vi "Test_ExecuteCalibration.vi"() -> ()   [LabVIEW 2019]
uses:
  ByteGSAPIBase/CalibrationMeasurements/BodyCalibrazioneMisure.ctl
  ByteGSAPIBase/FetchCalibration/Converted_Slug_Cluster.ctl
  ByteGSAPIBase/ByteGSAPIBase.lvclass
  <vilib>/DAQmx/write.llb/DAQmx Write (Analog DBL 1Chan 1Samp).vi
  <vilib>/DAQmx/read.llb/DAQmx Read (Analog DBL 1Chan 1Samp).vi
  2f0a0fb9-248b-477a-8bd2-6224b53458e2.vi
  <vilib>/DAQmx/create/channels.llb/DAQmx Create Channel (AI-Voltage-Basic).vi
  <vilib>/DAQmx/create/channels.llb/DAQmx Create Channel (AO-Voltage-Basic).vi
  <vilib>/DAQmx/miscellaneous.llb/DAQmx Fill In Error Info.vi
  <vilib>/Bytelabs/ByteSimpleQ/ByteSimpleQ/ByteSimpleQ.lvlib
panel:
  in  "Exit":bool
  in  "Calibrate":bool
  in  "Btn-Start-Oriz":bool
  in  "DueDateInstruments":i32(listbox)
  out "Waveform Chart":dbl(graph)
  out "logical AND":bool
  out "Mpe_min":dbl format="%.3f"
  out "Mpe_Max":dbl format="%.3f"
  out "Temp":sgl format="%.1f °C"
  out "Hr%":sgl format="%.1f Hr%"
  out "nmisure":u32 format="# %d"
  out "UoM":string
  out "Measure":dbl format="%0.2f"
  out "measurement_group_passed":u32(colorbox)
  in  "SetPoint":dbl format="%0.2f"
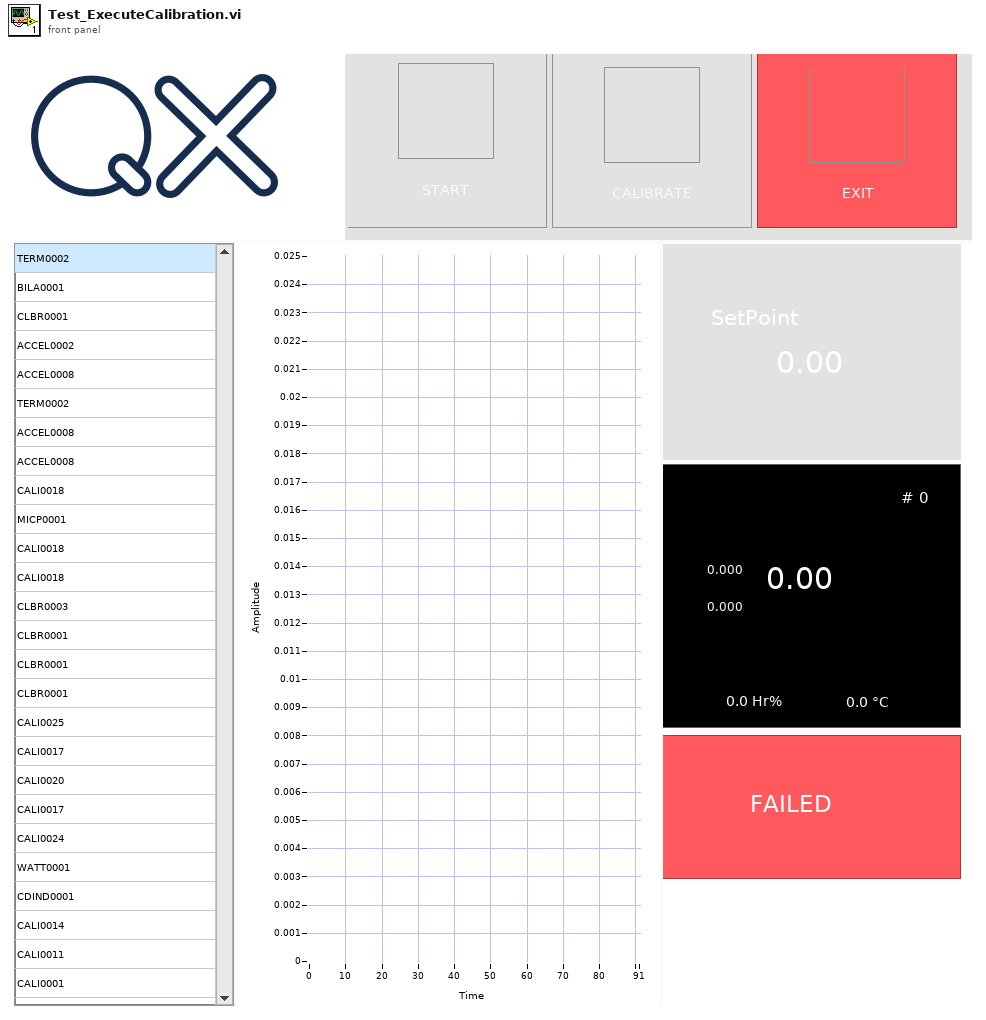
[diagram p1: front panel]
types:
  T1 = typedef "ByteGSWebAPI.lvlib/ByteGSAPIBase.lvclass/BodyCalibrazioneMisure.ctl" = cluster{"controls":cluster{"id":u16, "descrizione":string, "numero_misure_necessarie":u16, "riferimento_obiettivo":dbl, "mpe_max":dbl, "mpe_min":dbl, "deviazione_standard":dbl, "incertezza":dbl, "numero_misure_effettuate":u32, "temperatura_c":dbl, "umidita":dbl, "strumento_riferimento":cluster{"id":u16, "nome":string}[]}[]}
  T2 = typedef "ByteGSWebAPI.lvlib/ByteGSAPIBase.lvclass/Converted_Slug_Cluster.ctl" = cluster{"id":u32, "instrument":string, "name":string, "date":timestamp}
  T3 = cluster{"AI":refnum<k21>, "AO":refnum<k21>, "IdInstrument":i32[], "Calibration data":T1, "Measure":dbl, "idFailed":u32, "passed":bool, "Read?":bool, "CalibIndex":i32, "TotMeasure":i32, "riferimento_obiettivo":dbl, "ExpiredInstruments":T2[]}
  T4 = enum8{"Enabled", "Disabled", "Disabled and Grayed Out"}
  T5 = typedef "Instruments.ctl" = cluster{"id":i32, "slug":string, "stabilimento":cluster{"id":dbl}, "categoria":cluster{"id":dbl}, "tipologia_di_visualizzazione":cluster{"id":dbl}, "stato":cluster{"id":dbl}, "descrizione":string, "costruttore":string, "matricola":string, "data_registrazione":string, "intervallo_di_taratura_mesi":dbl, "reparto":string, "campo_misura":string, "risoluzione":dbl, "responsabile_strumento":string, "classe_di_precisione":string, "classificazione":string, "appunti":string, "manuale":string, "foto":string, "riferimento":bool, "qr_hashcode":string, "costo_euro":dbl}
  T6 = cluster{"id":u16, "descrizione":string, "numero_misure_necessarie":u16, "riferimento_obiettivo":dbl, "mpe_max":dbl, "mpe_min":dbl, "deviazione_standard":dbl, "incertezza":dbl, "numero_misure_effettuate":u32, "temperatura_c":dbl, "umidita":dbl, "strumento_riferimento":cluster{"id":u16, "nome":string}[]}[]
  T7 = cluster{"id":u16, "descrizione":string, "numero_misure_necessarie":u16, "riferimento_obiettivo":dbl, "mpe_max":dbl, "mpe_min":dbl, "deviazione_standard":dbl, "incertezza":dbl, "numero_misure_effettuate":u32, "temperatura_c":dbl, "umidita":dbl, "strumento_riferimento":cluster{"id":u16, "nome":string}[]}
  T8 = cluster{"id":u32, "control_id":u32, "passed":bool}[]
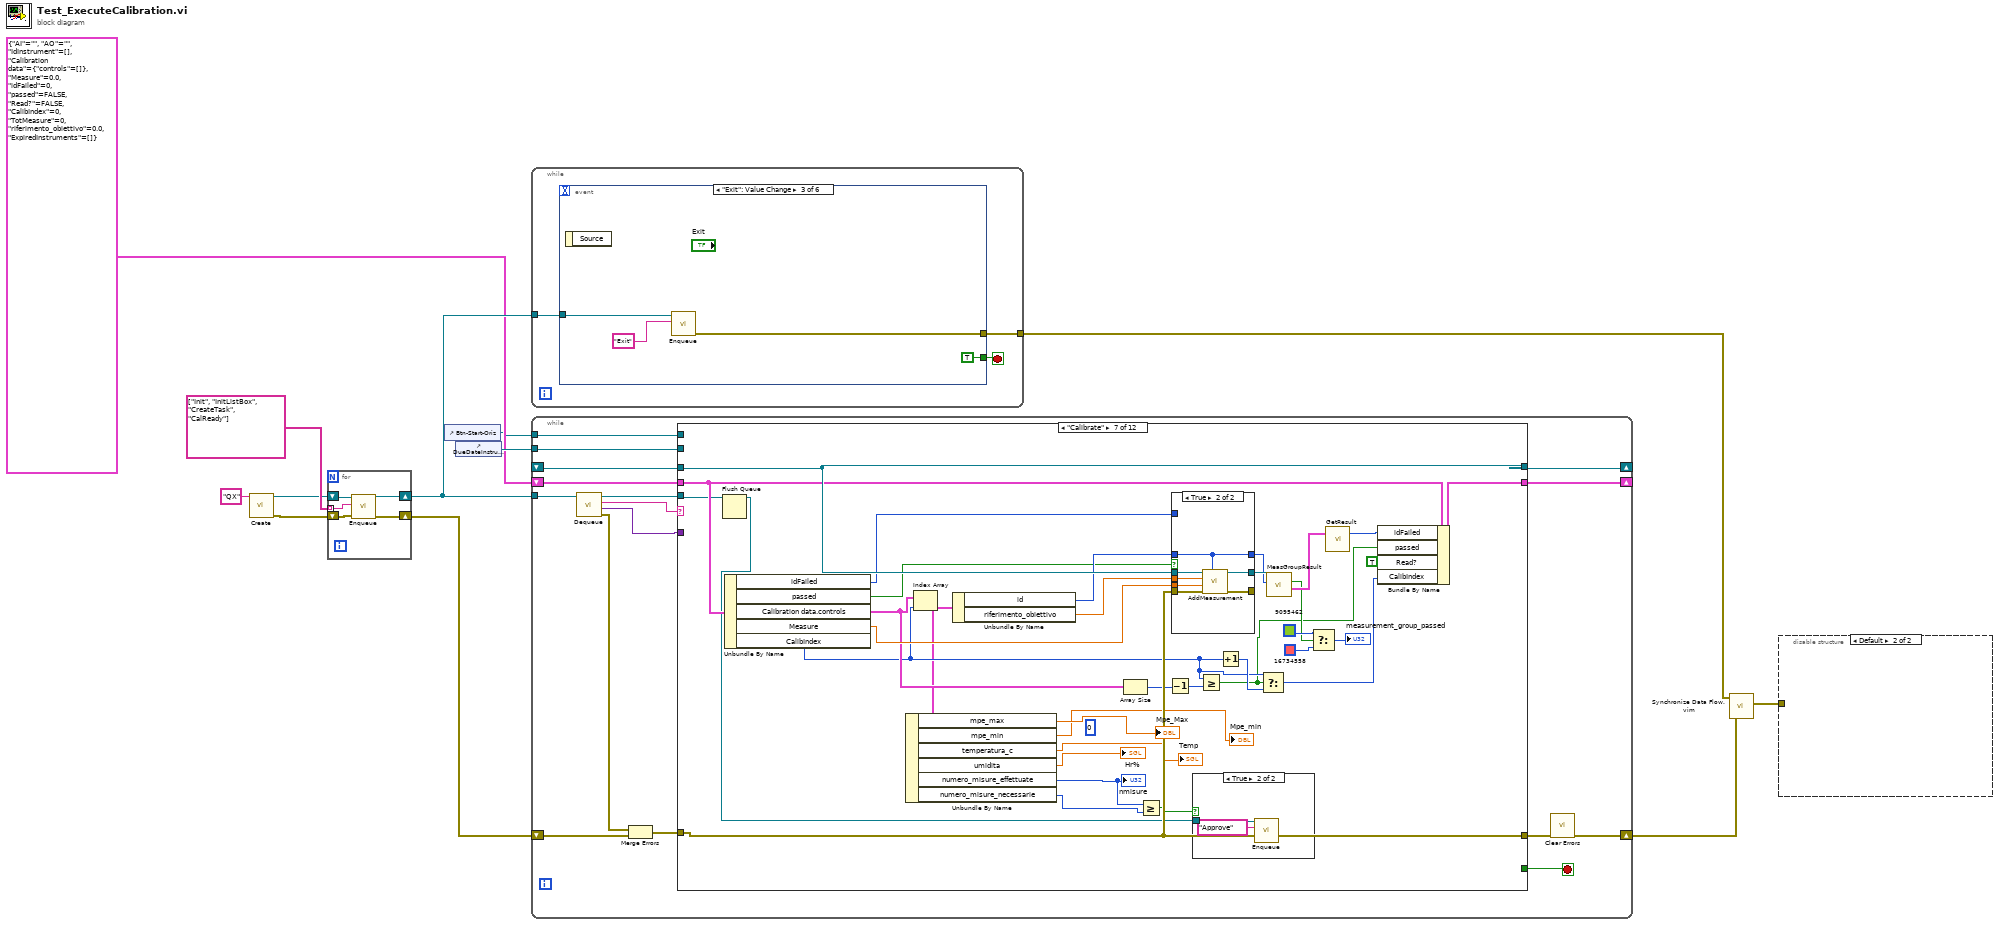
[diagram p0: block diagram]
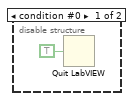
[diagram p2: hidden frame]
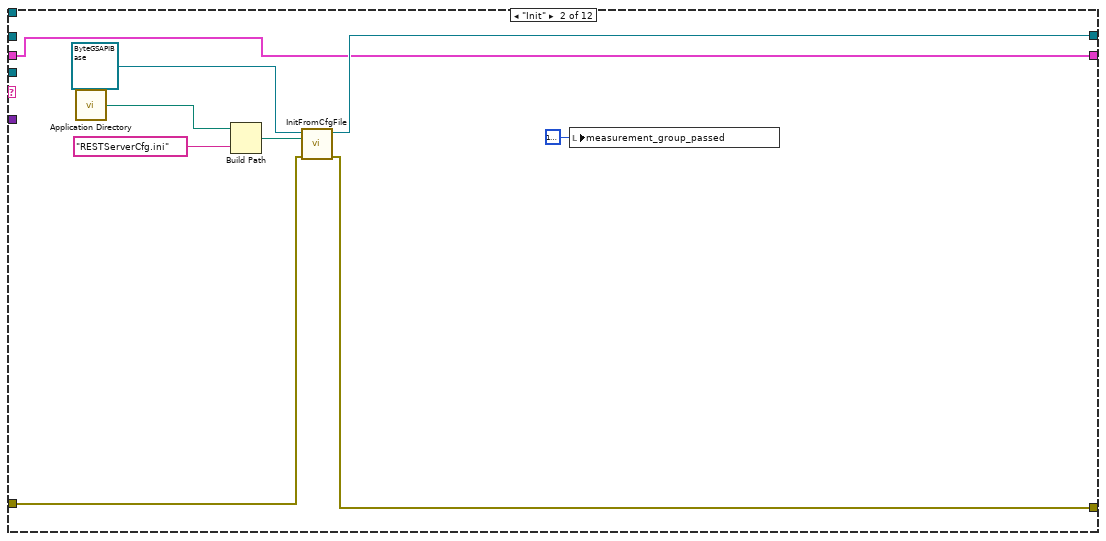
[diagram p4: hidden frame]
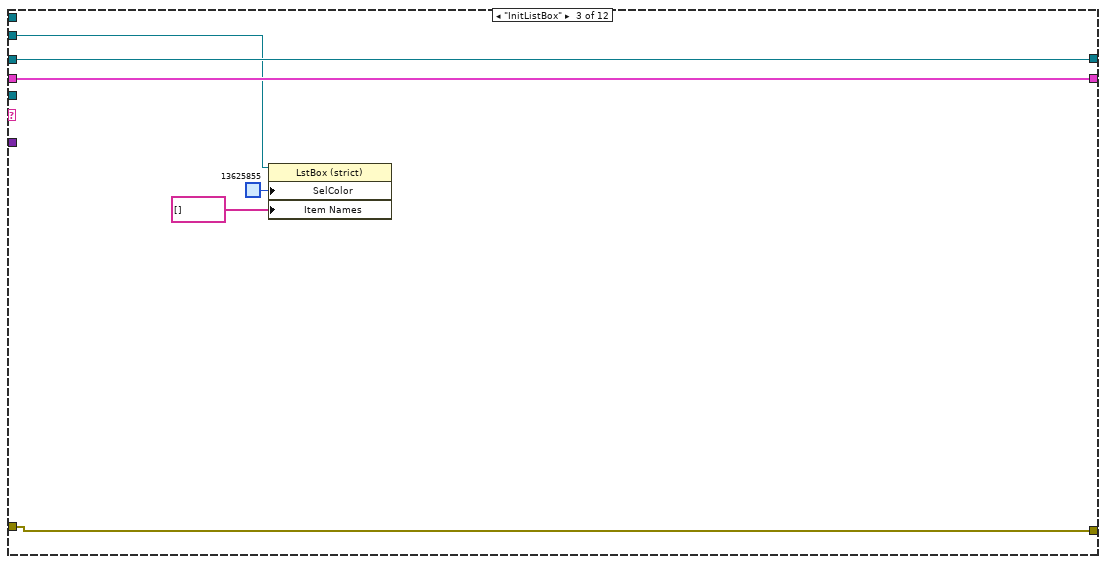
[diagram p5: hidden frame]
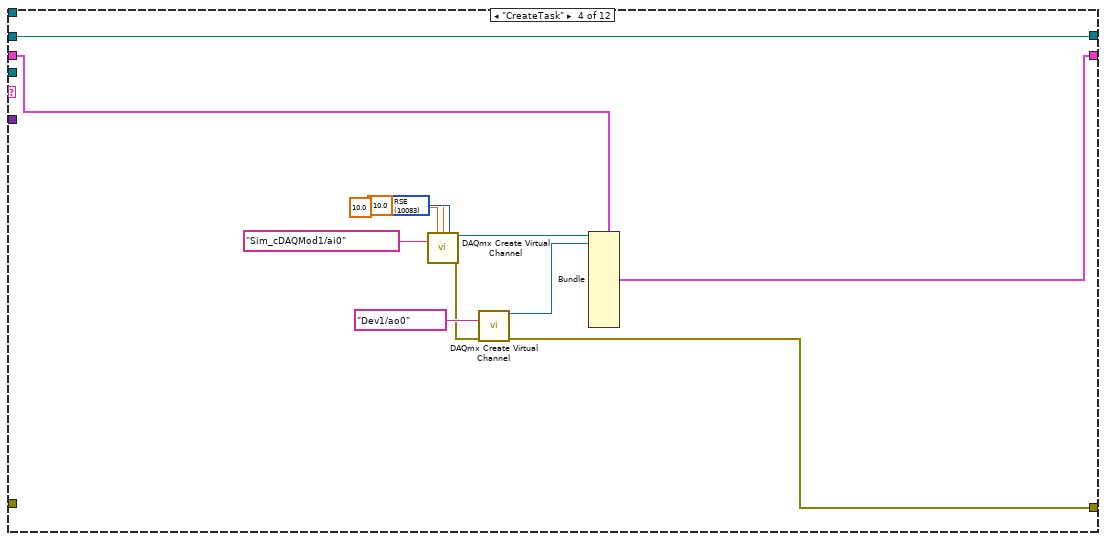
[diagram p6: hidden frame]
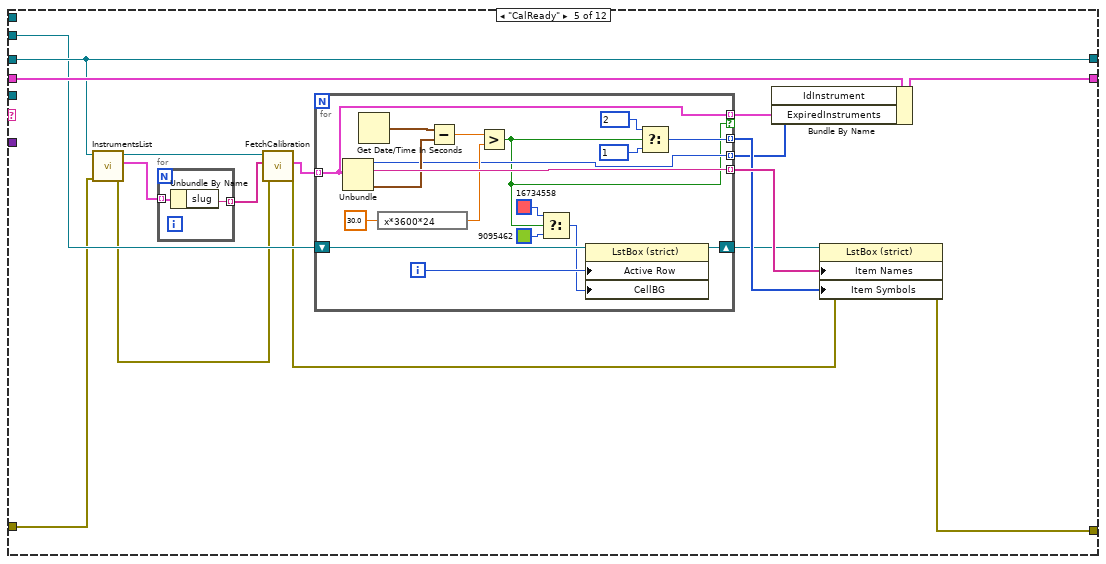
[diagram p7: hidden frame]
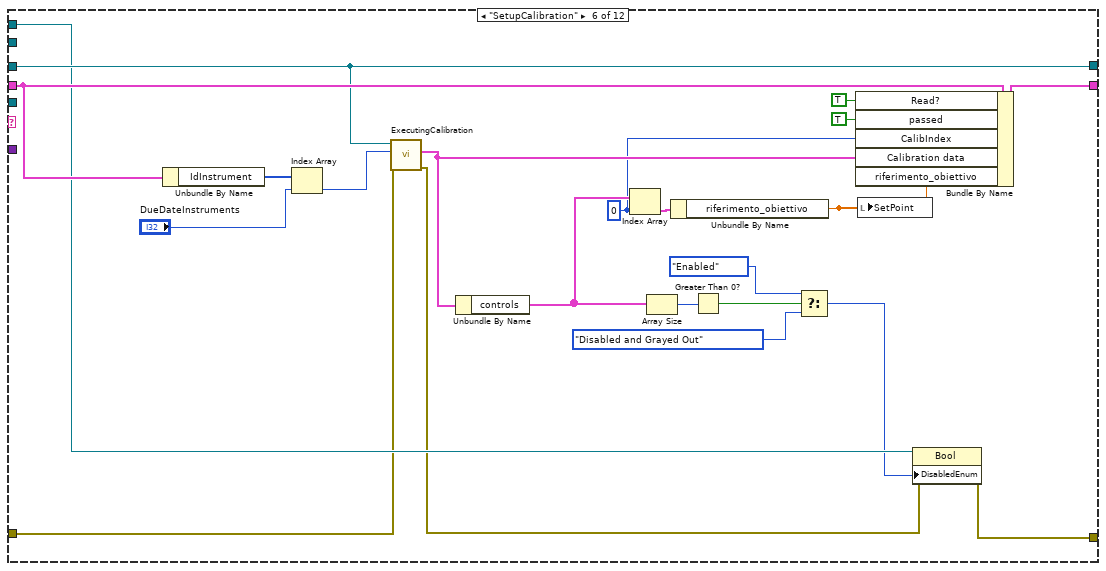
[diagram p8: hidden frame]
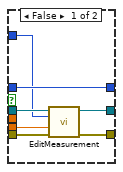
[diagram p10: hidden frame]
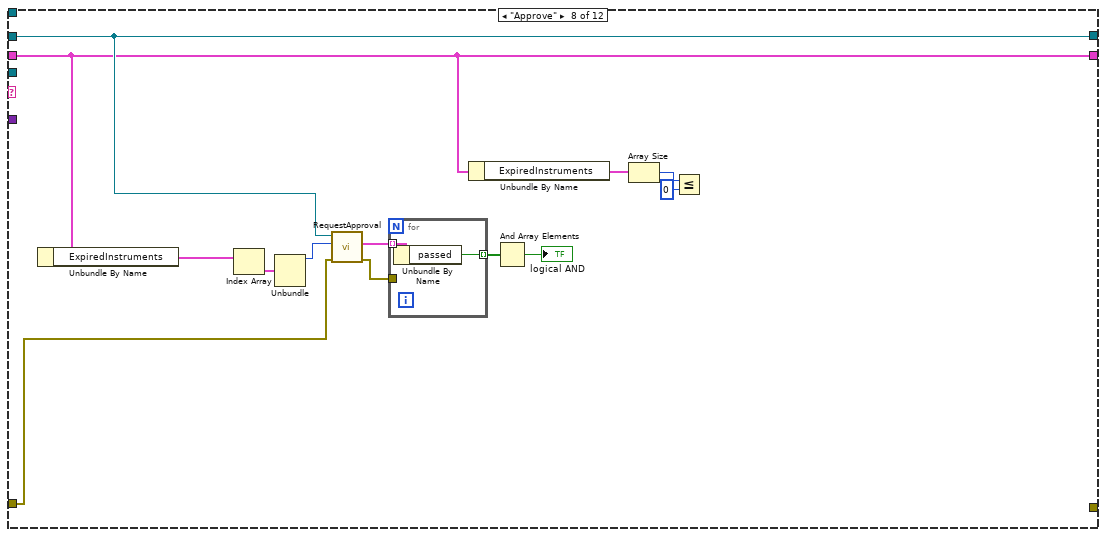
[diagram p11: hidden frame]
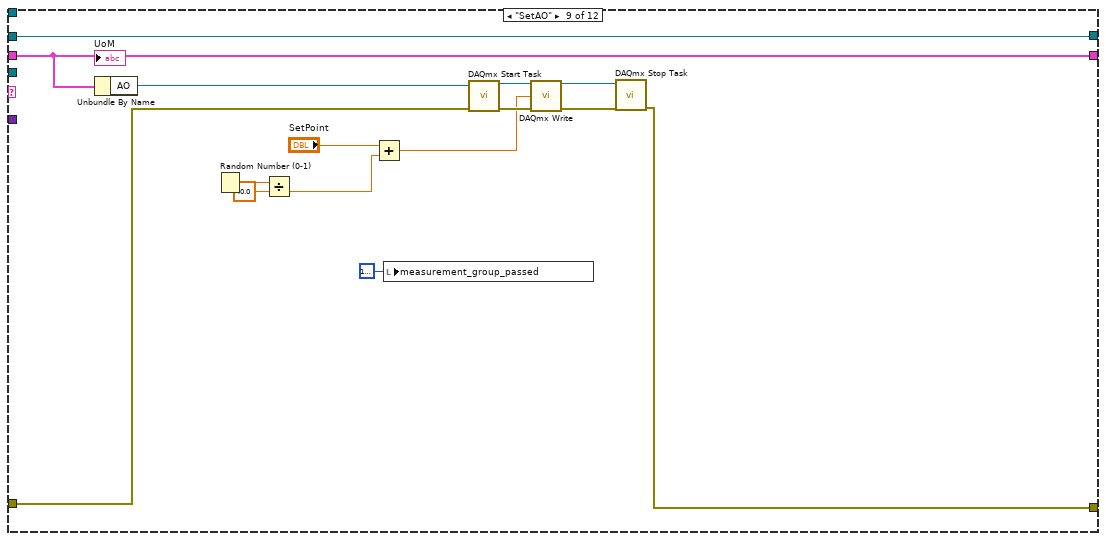
[diagram p12: hidden frame]
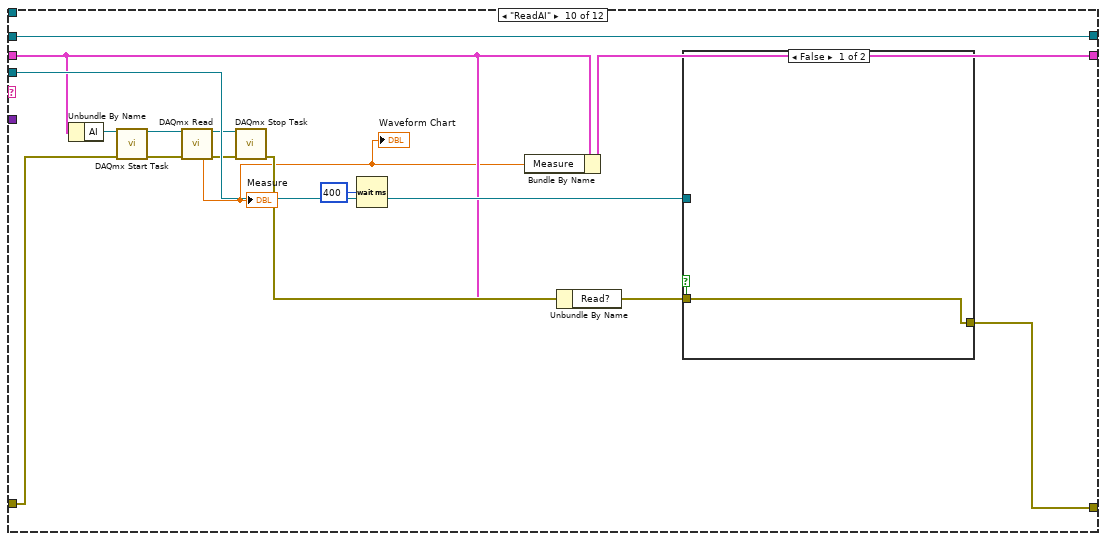
[diagram p13: hidden frame]
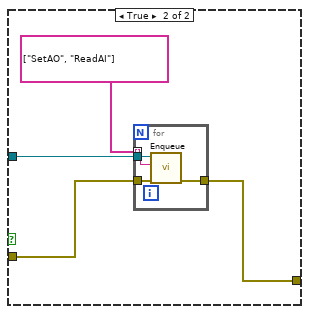
[diagram p14: hidden frame]
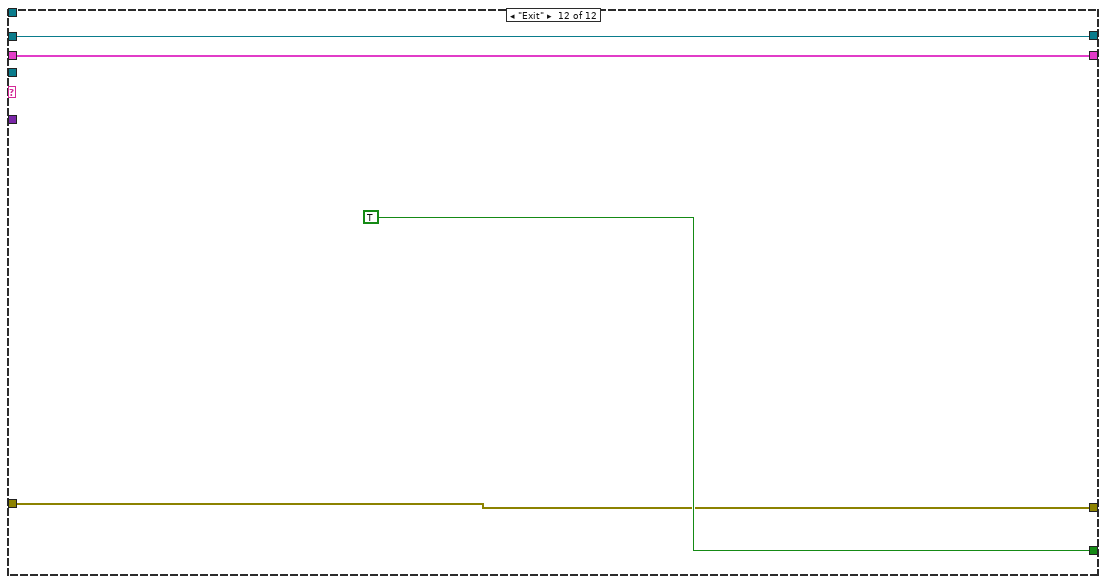
[diagram p16: hidden frame]
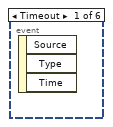
[diagram p17: hidden frame]
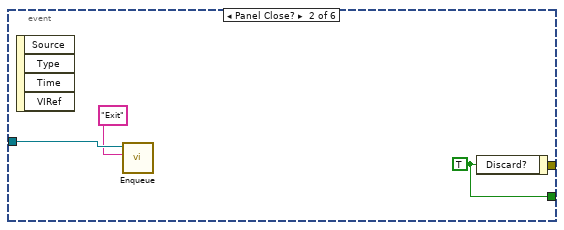
[diagram p18: hidden frame]
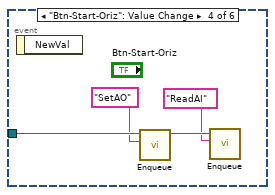
[diagram p19: hidden frame]
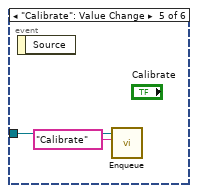
[diagram p20: hidden frame]
diagram:
  n1 = call <vilib>:"Create.vi"("name (unnamed)"="QX") -> ("error out"=w9:errorcluster, "queue out"=w10:refnum<queue>)  [unwired: 8 in, 1 out]
  n2 = for {
    tunnel: string[] ["Init", "InitListBox", "CreateTask", "CalReady"] ("message") -> [w17] mode=indexing
    shift-right: [w15] -> w8
    shift-left: w10 -> [w16]
    shift-right: [w13] -> w7
    shift-left: w9 -> [w14]
    n3 = call <vilib>:"Enqueue.vi"("error in (no error)"=w14, "message"=w17, "queue in"=w16) -> ("error out"=w13:errorcluster, "queue out"=w15:refnum<queue>)  [unwired: 6 in, 1 out]
  }
  n4 = control-ref of="Btn-Start-Oriz"() -> (w4:refnum<vi>)
  n5 = control-ref of="DueDateInstruments"() -> (w6:refnum<vi>)
  n6 = while {
    tunnel: w8 -> [w19]
    tunnel: [w18] -> w2
    stop <- w20 stop-if-true
    n7 = event shown="[2] \"Exit\": Value Change" {
      selector: _ -> [_ _ _ _ _ _]
      dyn-events: _ -> [_ _ _ _ _ _]
      timeout: _ -> [_ _ _ _ _ _]
      tunnel: [_ w23 TRUE ("Discard?") _ _ _] -> w20
      tunnel: w19 -> [_ w22 w26 w31 w33 w35]
      tunnel: [_ _ w25 _ _ _] -> w18
      event Timeout {
        n8 = event-data() -> ()  [unwired: 1 in, 3 out]
      }
      event Panel Close? {
        w23 = TRUE ("Discard?")
        n9 = event-data() -> ()  [unwired: 1 in, 4 out]
        n10 = call <vilib>:"Enqueue.vi"("message"="Exit", "queue in"=w22) -> ()  [unwired: 7 in, 3 out]
        n11 = event-data("Discard?"=w23) -> ()  [unwired: 1 in, 1 out]
      }
      event "Exit": Value Change {
        n12 = event-data() -> ()  [unwired: 1 in, 1 out]
        n13 = call <vilib>:"Enqueue.vi"("message"="Exit", "queue in"=w26) -> ("error out"=w25:errorcluster)  [unwired: 7 in, 2 out]
      }
      event "Btn-Start-Oriz": Value Change {
        n14 = event-data() -> ()  [unwired: 1 in, 1 out]
        n15 = call <vilib>:"Enqueue.vi"("message"="SetAO", "queue in"=w31) -> ("queue out"=w29:refnum<queue>)  [unwired: 7 in, 2 out]
        n16 = call <vilib>:"Enqueue.vi"("message"="ReadAI", "queue in"=w29) -> ()  [unwired: 7 in, 3 out]
      }
      event "Calibrate": Value Change {
        n17 = event-data() -> ()  [unwired: 1 in, 1 out]
        n18 = call <vilib>:"Enqueue.vi"("message"="Calibrate", "queue in"=w33) -> ()  [unwired: 7 in, 3 out]
      }
      event "DueDateInstruments": Double Click {
        n19 = event-data() -> ()  [unwired: 1 in, 1 out]
        n20 = call <vilib>:"Enqueue.vi"("message"="SetupCalibration", "queue in"=w35) -> ()  [unwired: 7 in, 3 out]
      }
    }
  }
  n21 = while {
    tunnel: w8 -> [w50]
    shift-right: [w36] -> w3
    shift-left: w7 -> [w44]
    shift-right: [w43] -> _
    shift-left: _ -> [w42]
    shift-right: [w41] -> _
    shift-left: T3 {"AI"="", "AO"="", "IdInstrument"=[], "Calibration data"={"controls"=[]}, "Measure"=0.0, "idFailed"=0, "passed"=FALSE, "Read?"=FALSE, "CalibIndex"=0, "TotMeasure"=0, "riferimento_obiettivo"=0.0, "ExpiredInstruments"=[]} ("output cluster") -> [w40]
    tunnel: w6 -> [w38]
    tunnel: w4 -> [w37]
    stop <- w51 stop-if-true
    n22 = call <vilib>:"Dequeue.vi"("queue in"=w50) -> ("error out"=w46:errorcluster, "data"=w47:variant, "message"=w48:string, "queue out"=w49:refnum<queue>)  [unwired: 6 in, 1 out]
    n23 = Merge Errors(w46, w44) -> (w45:errorcluster)
    n24 = case shown="\"Calibrate\"" w48 {
      tunnel: [_ _ _ _ _ _ _ _ _ _ _ TRUE] -> w51
      tunnel: w49 -> [_ _ _ _ _ _ w162 _ _ w234 _ _]
      tunnel: w47 -> [_ _ _ _ _ _ _ _ _ _ _ _]
      tunnel: w45 -> [w54 w59 w69 _ w87 w121 w169 w200 w213 w230 w248 w251]
      tunnel: [w54 w58 w69 w75 w88 w119 w169 _ w214 w233 w248 w251] -> w39
      tunnel: [w53 w57 w68 w81 w97 w137 w174 w202 w221 w236 w247 w250] -> w43
      tunnel: w42 -> [w53 _ w68 w81 w97 w137 w174 w202 w221 w236 w247 w250]
      tunnel: [w52 w56 w67 w77 w84 w135 w166 w199 w211 w225 w246 w249] -> w41
      tunnel: w40 -> [w52 w56 w67 w70 w98 w140 w172 w199 w211 w224 w246 w249]
      tunnel: w38 -> [_ _ w66 _ w90 _ _ _ _ _ _ _]
      tunnel: w37 -> [_ _ _ _ _ w132 _ _ _ _ _ _]
      frame Default {
      }
      frame "Init" {
        n25 = call <vilib>:"Application Directory.vi"() -> ("Application Directory"=w62:path)
        n26 = Build Path(base path=w62, name or relative path="RESTServerCfg.ini") -> (appended path=w61:path)
        n27 = call-dynamic "InitFromCfgFile.vi"("error in (no error)"=w59, "configuration file path"=w61, "ByteGSAPIBase in"=refnum<class "ByteGSAPIBase.lvclass"> refnum) -> ("error out"=w58:errorcluster, "ByteGSAPIBase out"=w57:refnum<class "ByteGSAPIBase.lvclass">)  [unwired: 7 in]
        n28 = local write "measurement_group_passed"(u32 16777224 ("measurement_group_passed")) -> ()
      }
      frame "InitListBox" {
        n29 = property class="LstBox (strict)"(reference=w66, "SelColor"=u32 13625855 ("Selection Color"), "Item Names"=string[] []) -> ()  [unwired: 1 in, 2 out]
      }
      frame "CreateTask" {
        w73 = 10083 items=["Default"=-1, "RSE"=10083, "NRSE"=10078, "Differential"=10106, "Pseudodifferential"=12529] ("input terminal configuration")
        n30 = call-poly <vilib>:"DAQmx Create Virtual Channel.vi"("maximum value"=10.0, "minimum value"=-10.0, "input terminal configuration"=w73, "physical channels"=tag "Sim_cDAQMod1/ai0") -> ("task out"=w76:refnum<k21>, "error out"=w74:errorcluster)  [unwired: 10 in]
        n31 = call-poly <vilib>:"DAQmx Create Virtual Channel.vi"("physical channels"=tag "Dev1/ao0", "error in"=w74) -> ("task out"=w78:refnum<k21>, "error out"=w75:errorcluster)  [unwired: 12 in]
        n32 = Bundle(cluster=w70, "AI"=w76, "AO"=w78) -> (w77:T3)  [unwired: 10 in]
      }
      frame "CalReady" {
        n33 = call "InstrumentsList.vi"("error in (no error)"=w87, "ByteGSAPIBase in"=w97) -> ("error out"=w86:errorcluster, "Array"=w95:T5[], "ByteGSAPIBase out"=w96:refnum<class "ByteGSAPIBase.lvclass">)  [unwired: 7 in]
        n34 = for {
          tunnel: w95 -> [w118] mode=indexing
          tunnel: [w117] -> w94 mode=indexing
          n35 = Unbundle By Name(w118) -> ("slug"=w117:string)
        }
        n36 = call "FetchCalibration.vi"("error in (no error)"=w86, "Instruments"=w94, "ByteGSAPIBase in"=w96) -> ("error out"=w85:errorcluster, "Instruments"=w93:T2[])  [unwired: 6 in, 1 out]
        n37 = for {
          tunnel: w93 -> [w100] mode=indexing
          tunnel: [w116] -> w92 mode=indexing
          tunnel: [w108] -> w91 mode=indexing
          shift-right: [w102] -> w89
          shift-left: w90 -> [w106]
          tunnel: [w101] -> w83 mode=indexing
          tunnel: [w100] -> w82 mode=indexing if=w99
          i -> [w107]
          n38 = Unbundle(w100) -> ("id"=w101:u32, "instrument"=w116:string, "date"=w114:timestamp)  [unwired: 1 out]
          n39 = Get Date/Time In Seconds() -> (seconds since 1Jan1904=w115:timestamp)
          n40 = expression code="x*3600*24"(30.0 ("y")) -> (w112:dbl)
          n41 = Subtract(x=w115, y=w114) -> (x-y=w113:dbl)
          n42 = Greater?(x=w113, y=w112) -> (0:w99:bool)
          n43 = Select(t=u32 16734558, s=w99, f=u32 9095462) -> (s? t:f=w104:u32)
          n44 = property class="LstBox (strict)"(reference=w106, "Active Row"=w107, "CellBG"=w104) -> (reference out=w102:refnum<vi>)  [unwired: 1 in, 1 out]
          n45 = Select(t=2, s=w99, f=1) -> (s? t:f=w108:i32)
        }
        n46 = Bundle By Name(cluster=w98, "IdInstrument"=w83, "ExpiredInstruments"=w82) -> (w84:T3)
        n47 = property class="LstBox (strict)"(reference=w89, error in=w85, "Item Names"=w92, "Item Symbols"=w91) -> (error out=w88:errorcluster)  [unwired: 1 out]
      }
      frame "SetupCalibration" {
        w124 = 0 ("index")
        n48 = Unbundle By Name(w140) -> ("IdInstrument"=w139:i32[])
        n49 = Index Array(array=w139, index="DueDateInstruments") -> (element=w136:i32)
        n50 = call "ExecutingCalibration.vi"("error in (no error)"=w121, "calibration_id"=w136, "ByteGSAPIBase in"=w137) -> ("error out"=w120:errorcluster, "Calibration data"=w134:T1)  [unwired: 6 in, 1 out]
        n51 = Unbundle By Name(w134) -> ("controls"=w127:T6)
        n52 = Index Array(array=w127, index=w124) -> (element=w126:T7)
        n53 = Array Size(array=w127) -> (size(s)=w133:i32)
        n54 = Unbundle By Name(w126) -> ("riferimento_obiettivo"=w125:dbl)
        n55 = Greater Than 0?(x=w133) -> (x > 0?=w131:bool)
        n56 = Select(t=T4."Enabled" ("Disabled"), s=w131, f=T4."Disabled and Grayed Out") -> (s? t:f=w129:T4)
        n57 = Bundle By Name(cluster=w140, "Read?"=TRUE, "passed"=TRUE, "CalibIndex"=w124, "Calibration data"=w134, "riferimento_obiettivo"=w125) -> (w135:T3)
        n58 = local write "SetPoint"(w125) -> ()
        n59 = property class="Bool"(reference=w132, error in=w120, "DisabledEnum"=w129) -> (error out=w119:errorcluster)  [unwired: 1 out]
      }
      frame "Calibrate" {
        (unwired) u32 0 ("nmisure")
        n60 = Flush Queue(queue=w162) -> (queue out=w142:refnum<queue>)  [unwired: 1 in, 2 out]
        n61 = Unbundle By Name(w172) -> ("idFailed"=w164:u32, "passed"=w163:bool, "Calibration data.controls"=w156:T6, "Measure"=w168:dbl, "CalibIndex"=w153:i32)
        n62 = Index Array(array=w156, index=w153) -> (element=w150:T7)
        n63 = Unbundle By Name(w150) -> ("mpe_max"=→"Mpe_Max":dbl, "mpe_min"=→"Mpe_min":dbl, "temperatura_c"=→"Temp":dbl, "umidita"=→"Hr%":dbl, "numero_misure_effettuate"=w145:u32, "numero_misure_necessarie"=w144:u16)
        "nmisure" <- w145
        n64 = Unbundle By Name(w150) -> ("id"=w171:u16, "riferimento_obiettivo"=w170:dbl)
        n65 = Array Size(array=w156) -> (size(s)=w155:i32)
        n66 = Greater Or Equal?(x=w145, y=w144) -> (x >= y?=w143:bool)
        n67 = Decrement(x=w155) -> (x-1=w151:i32)
        n68 = case shown="True" w163 {
          tunnel: w174 -> [w184 w191]
          tunnel: w170 -> [_ w190]
          tunnel: w168 -> [w182 w189]
          tunnel: w169 -> [w183 w188]
          tunnel: [w180 w187] -> _
          tunnel: w171 -> [w179 w185]
          tunnel: [w181 w186] -> w175
          tunnel: [w179 w185] -> w173
          tunnel: w164 -> [w178 _]
          frame False {
            n69 = call-dynamic "EditMeasurement.vi"("error in (no error)"=w183, "instrument measure"=w182, "measurement id"=w178, "ByteGSAPIBase in"=w184) -> ("error out"=w180:errorcluster, "ByteGSAPIBase out"=w181:refnum<class "ByteGSAPIBase.lvclass">)  [unwired: 5 in, 1 out]
          }
          frame True {
            n70 = call-dynamic "AddMeasurement.vi"("measurement_group id"=w185, "error in (no error)"=w188, "misura_strumento"=w189, "misura_riferimento"=w190, "ByteGSAPIBase in"=w191) -> ("error out"=w187:errorcluster, "ByteGSAPIBase out"=w186:refnum<class "ByteGSAPIBase.lvclass">)  [unwired: 4 in, 1 out]
          }
        }
        n71 = case shown="True" w143 {
          tunnel: w142 -> [_ w177]
          frame False {
          }
          frame True {
            n72 = call <vilib>:"Enqueue.vi"("message"="Approve", "queue in"=w177) -> ()  [unwired: 7 in, 3 out]
          }
        }
        n73 = Greater Or Equal?(x=w153, y=w151) -> (x >= y?=w141:bool)
        n74 = Increment(x=w153) -> (x+1=w154:i32)
        n75 = Select(t=w153, s=w141, f=w154) -> (s? t:f=w152:i32)
        n76 = call "MeasGroupResult.vi"("measurement_group_id"=w173, "ByteGSAPIBase in"=w175) -> ("measurements"=w167:cluster{"id":u32, "passed":bool}[], "measurement_group_passed"=w158:bool)  [unwired: 6 in, 2 out]
        n77 = Select(t=u32 9095462 ("measurement_group_passed"), s=w158, f=u32 16734558 ("measurement_group_passed")) -> (s? t:f=→"measurement_group_passed":u32)
        n78 = call "GetResult.vi"("measurements"=w167) -> ("id"=w165:u32)  [unwired: 1 in, 1 out]
        n79 = Bundle By Name(cluster=w172, "idFailed"=w165, "passed"=w141, "Read?"=TRUE, "CalibIndex"=w152) -> (w166:T3)
      }
      frame "Approve" {
        n80 = Unbundle By Name(w199) -> ("ExpiredInstruments"=w201:T2[])
        n81 = Index Array(array=w201) -> (element=w204:T2)  [unwired: 1 in]
        n82 = Unbundle(w204) -> ("id"=w203:u32)  [unwired: 3 out]
        n83 = call "RequestApproval.vi"("error in (no error)"=w200, "calibration_id"=w203, "ByteGSAPIBase in"=w202) -> ("error out"=w192:errorcluster, "controls"=w195:T8)  [unwired: 6 in, 1 out]
        n84 = for {
          tunnel: w195 -> [w206] mode=indexing
          tunnel: [w205] -> w194 mode=indexing
          tunnel: w192 -> [_]
          n85 = Unbundle By Name(w206) -> ("passed"=w205:bool)
        }
        n86 = Unbundle By Name(w199) -> ("ExpiredInstruments"=w198:T2[])
        n87 = And Array Elements(Boolean array=w194) -> (logical AND=→"logical AND":bool)
        n88 = Array Size(array=w198) -> (size(s)=w197:i32)
        n89 = Less Or Equal?(x=w197, y=0) -> ()  [unwired: 1 out]
      }
      frame "SetAO" {
        n90 = Unbundle By Name(w211) -> ("AO"=w220:refnum<k21>)
        n91 = Random Number (0-1)() -> (number: 0 to 1=w208:dbl)
        n92 = Divide(x=w208, y=40.0) -> (x/y=w209:dbl)
        n93 = Add(x="SetPoint", y=w209) -> (x+y=w212:dbl)
        n94 = local write "measurement_group_passed"(u32 16777224 ("measurement_group_passed")) -> ()
        n95 = call <vilib>:"DAQmx Start Task.vi"("task/channels in"=w220, "error in"=w213) -> ("task out"=w218:refnum<k21>, "error out"=w217:errorcluster)  [unwired: 12 in]
        n96 = call-poly <vilib>:"DAQmx Write.vi"("task/channels in"=w218, "data"=w212, "error in"=w217) -> ("task out"=w216:refnum<k21>, "error out"=w215:errorcluster)  [unwired: 10 in, 1 out]
        n97 = call <vilib>:"DAQmx Stop Task.vi"("task/channels in"=w216, "error in"=w215) -> ("error out"=w214:errorcluster)  [unwired: 12 in, 1 out]
      }
      frame "ReadAI" {
        n98 = Unbundle By Name(w224) -> ("AI"=w235:refnum<k21>)
        n99 = call <vilib>:"DAQmx Start Task.vi"("task/channels in"=w235, "error in"=w230) -> ("task out"=w231:refnum<k21>, "error out"=w229:errorcluster)  [unwired: 12 in]
        n100 = call-poly <vilib>:"DAQmx Read.vi"("task/channels in"=w231, "error in"=w229) -> ("task out"=w228:refnum<k21>, "data"=w222:dbl, "error out"=w227:errorcluster)  [unwired: 11 in]
        "Measure" <- w222
        "Waveform Chart" <- w222
        n101 = call <vilib>:"DAQmx Stop Task.vi"("task/channels in"=w228, "error in"=w227) -> ("error out"=w226:errorcluster)  [unwired: 12 in, 1 out]
        n102 = Wait (ms)(milliseconds to wait=u32 400) -> ()  [unwired: 1 out]
        n103 = Bundle By Name(cluster=w224, "Measure"=w222) -> (w225:T3)
        n104 = Unbundle By Name(w224) -> ("Read?"=w223:bool)
        n105 = case shown="False" w223 {
          tunnel: w234 -> [_ w240]
          tunnel: [w237 w239] -> w233
          tunnel: w226 -> [w237 w238]
          frame False {
          }
          frame True {
            n106 = for {
              tunnel: string[] ["SetAO", "ReadAI"] ("message") -> [w245] mode=indexing
              tunnel: w240 -> [w244]
              tunnel: [w243] -> w239
              tunnel: w238 -> [w242]
              n107 = call <vilib>:"Enqueue.vi"("error in (no error)"=w242, "message"=w245, "queue in"=w244) -> ("error out"=w243:errorcluster)  [unwired: 6 in, 2 out]
            }
          }
        }
      }
      frame "Idle" {
      }
      frame "Exit" {
      }
    }
    n108 = call <vilib>:"Clear Errors.vi"("error in (no error)"=w39) -> ("error out"=w36:errorcluster)  [unwired: 5 in, 1 out]
  }
  n109 = call "Synchronize Data Flow.vim"("input 2"=w3, "input 1"=w2) -> ("output 2"=w1:errorcluster)  [unwired: 2 in, 3 out]
  n110 = disable-structure shown="Default" {
    disable-tunnel: w1 -> [_ _]
    frame condition #0 {
      n111 = Quit LabVIEW(quit? (T)=TRUE) -> ()
    }
    frame condition #1 (active) {
    }
  }
